vi "FF+FB control (Rev.2).vi"() -> ()   [LabVIEW 2010]
uses:
  <vilib>/DAQmx/read.llb/DAQmx Read (Analog 1D DBL NChan 1Samp).vi
  <vilib>/DAQmx/write.llb/DAQmx Write (Analog DBL 1Chan 1Samp).vi
  <vilib>/DAQmx/create/channels.llb/DAQmx Create Channel (AI-Voltage-Basic).vi
  <vilib>/DAQmx/configure/timing.llb/DAQmx Timing (Sample Clock).vi
  <vilib>/DAQmx/create/channels.llb/DAQmx Create Channel (AO-Voltage-Basic).vi
  <vilib>/daqmx/miscellaneous.llb/DAQmx Fill In Error Info.vi
panel:
  in  "ch2-1估測DC時間(秒)":dbl=1.0
  in  "ch2-2 估測DC時間(秒)":dbl=0.75
  in  "ch2 Kii 增益":dbl=-60000.0
  in  "ch2 Kp 增益":dbl
  out "overload":bool
  in  "ch1 Kp 增益":dbl=-250.0
  in  "ch2 Ki 增益":dbl=-83.5
  in  "ch1 Ki 增益":dbl=-10000.0
  in  "ch1-2估測DC時間(秒)":dbl=1.0
  in  "ch2-3估測DC時間(秒)":dbl=0.5
  in  "Controller on":bool
  out "error out":errorcluster
  out "延遲百分比(%)  需小於0.5%":dbl=0.3028175195295191
  out "理想迴圈時間(ms)":dbl=0.14285714285714288
  out "迴圈平均運行時間(ms)":dbl=0.14328973931361363
  in  "output channels 1":tag="PXI-6733/ao0"
  in  "stop":bool
  in  "ch1-1估測DC時間(秒)":dbl=2.0
  in  "每通道取樣頻率(Hz)":dbl=7000.0 format="%0.2f"
  in  "input channels 2":tag="PXI-6229/ai1"
  in  "input channels 1":tag="PXI-6229/ai0"
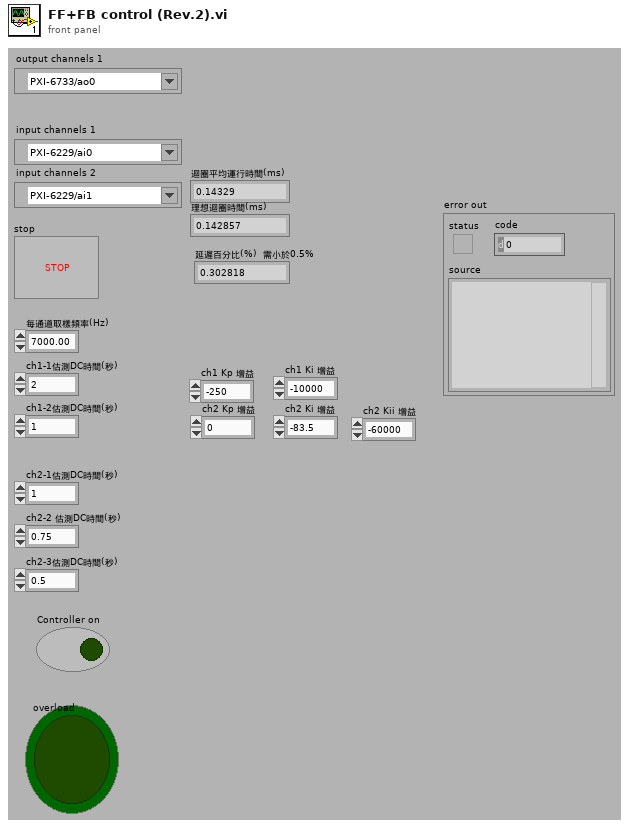
[diagram p1: front panel]
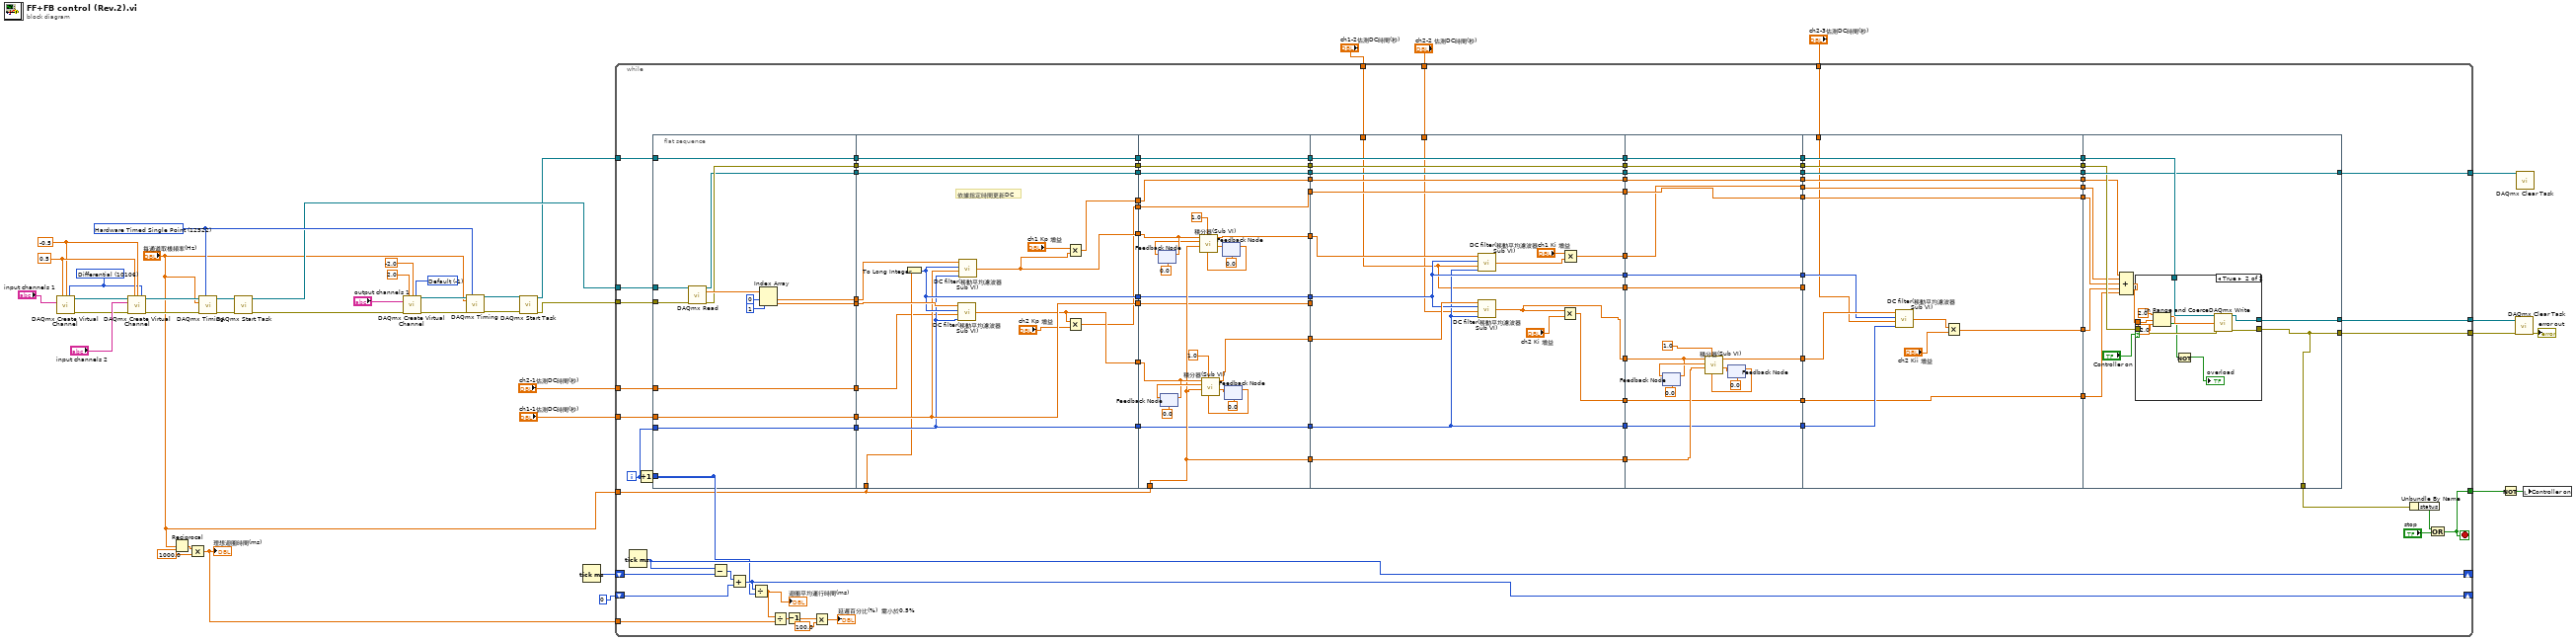
[diagram p0: block diagram]
diagram:
  w28 = -1 items=["Default"=-1, "RSE"=10083, "Differential"=10106, "Pseudodifferential"=12529] ("output terminal configuration")
  w25 = 12522 items=["Finite Samples"=10178, "Continuous Samples"=10123, "Hardware Timed Single Point"=12522] ("sample mode")
  w36 = 10106 items=["default"=-1, "RSE"=10083, "NRSE"=10078, "Differential"=10106, "Pseudodifferential"=12529] ("input terminal configuration")
  w37 = -0.5 ("minimum value")
  w38 = 0.5 ("maximum value")
  n1 = call-poly <vilib>:"DAQmx Create Virtual Channel.vi"("maximum value"=w38, "minimum value"=w37, "input terminal configuration"=w36, "physical channels"="input channels 1") -> ("task out"=w41:refnum<k21>, "error out"=w33:errorcluster)  [unwired: 10 in]
  n2 = call-poly <vilib>:"DAQmx Create Virtual Channel.vi"("task in"=w41, "maximum value"=w38, "minimum value"=w37, "input terminal configuration"=w36, "physical channels"="input channels 2", "error in"=w33) -> ("task out"=w35:refnum<k21>, "error out"=w32:errorcluster)  [unwired: 8 in]
  n3 = Reciprocal(x="每通道取樣頻率(Hz)") -> (1/x=w16:dbl)
  n4 = Multiply(x=w16, y=1000.0) -> (x*y=w14:dbl)
  "理想迴圈時間(ms)" <- w14
  n5 = call-poly <vilib>:"DAQmx Timing.vi"("task/channels in"=w35, "sample mode"=w25, "rate"="每通道取樣頻率(Hz)", "error in"=w32) -> ("task out"=w34:refnum<k21>, "error out"=w31:errorcluster)  [unwired: 10 in]
  n6 = call <vilib>:"DAQmx Start Task.vi"("task/channels in"=w34, "error in"=w31) -> ("task out"=w21:refnum<k21>, "error out"=w22:errorcluster)  [unwired: 12 in]
  n7 = call-poly <vilib>:"DAQmx Create Virtual Channel.vi"("maximum value"=2.0, "minimum value"=-2.0 ("maximum value"), "output terminal configuration"=w28, "physical channels"="output channels 1", "error in"=w22) -> ("task out"=w27:refnum<k21>, "error out"=w26:errorcluster)  [unwired: 9 in]
  n8 = call-poly <vilib>:"DAQmx Timing.vi"("task/channels in"=w27, "sample mode"=w25, "rate"="每通道取樣頻率(Hz)", "error in"=w26) -> ("task out"=w24:refnum<k21>, "error out"=w23:errorcluster)  [unwired: 10 in]
  n9 = call <vilib>:"DAQmx Start Task.vi"("task/channels in"=w24, "error in"=w23) -> ("task out"=w12:refnum<k21>, "error out"=w20:errorcluster)  [unwired: 12 in]
  n10 = Tick Count (ms)() -> (millisecond timer value=w18:u32)
  n11 = while {
    tunnel: w21 -> [w130]
    tunnel: w20 -> [w129]
    shift-right: [w125] -> _
    shift-left: w18 -> [w126]
    shift-right: [w122] -> _
    shift-left: 0 ("index") -> [w123]
    tunnel: w14 -> [w119]
    tunnel: "每通道取樣頻率(Hz)" -> [w69]
    tunnel: w12 -> [w106]
    tunnel: [w99] -> w9
    tunnel: [w67] -> w8
    tunnel: [w86] -> w7
    tunnel: "ch1-1估測DC時間(秒)" -> [w85]
    tunnel: [w68] -> w5
    tunnel: "ch1-2估測DC時間(秒)" -> [w46]
    tunnel: "ch2-3估測DC時間(秒)" -> [w45]
    tunnel: "ch2-2 估測DC時間(秒)" -> [w44]
    tunnel: "ch2-1估測DC時間(秒)" -> [w43]
    i -> [w83]
    stop <- w68 stop-if-true
    n12 = Tick Count (ms)() -> (millisecond timer value=w125:u32)
    n13 = Increment(x=w83) -> (x+1=w121:i32)
    n14 = flat-sequence {
      tunnel: w130 -> [w143]
      tunnel: w129 -> [w142]
      tunnel: [w138] -> w128
      tunnel: [w137] -> w127
      tunnel: w121 -> [_]
      tunnel: w106 -> [w136]
      tunnel: [w136] -> w100
      tunnel: [w135] -> w98
      tunnel: [w134] -> w92
      tunnel: w85 -> [w133]
      tunnel: [w133] -> w84
      tunnel: w83 -> [w132]
      tunnel: [w132] -> w82
      tunnel: w43 -> [w131]
      tunnel: [w131] -> w42
      tunnel: w128 -> [w156]
      tunnel: w127 -> [w155]
      tunnel: [w146] -> w114
      tunnel: [w149] -> w113
      tunnel: [w159] -> w101
      tunnel: w100 -> [w159]
      tunnel: w98 -> [w158]
      tunnel: [w158] -> w97
      tunnel: w92 -> [w157]
      tunnel: [w157] -> w87
      tunnel: w84 -> [w153]
      tunnel: w82 -> [w152]
      tunnel: [w154] -> w80
      tunnel: [w153] -> w79
      tunnel: [w152] -> w76
      tunnel: w69 -> [w151]
      tunnel: [w148] -> w59
      tunnel: [w145] -> w54
      tunnel: w42 -> [w144]
      tunnel: w114 -> [w173]
      tunnel: w113 -> [w184]
      tunnel: w69 -> [w170]
      tunnel: [w172] -> w112
      tunnel: [w171] -> w111
      tunnel: [w170] -> w108
      tunnel: [w169] -> w102
      tunnel: w101 -> [w169]
      tunnel: w97 -> [w168]
      tunnel: [w168] -> w95
      tunnel: [w167] -> w88
      tunnel: w87 -> [w167]
      tunnel: [w166] -> w81
      tunnel: w80 -> [w166]
      tunnel: w79 -> [w165]
      tunnel: [w165] -> w78
      tunnel: [w164] -> w77
      tunnel: w76 -> [w164]
      tunnel: w59 -> [w161]
      tunnel: [w161] -> w55
      tunnel: w54 -> [w160]
      tunnel: [w160] -> w53
      tunnel: w112 -> [w198]
      tunnel: w111 -> [w197]
      tunnel: [w190] -> w110
      tunnel: [w202] -> w109
      tunnel: w108 -> [w202]
      tunnel: [w201] -> w103
      tunnel: w102 -> [w201]
      tunnel: [w200] -> w96
      tunnel: w95 -> [w200]
      tunnel: [w199] -> w89
      tunnel: w88 -> [w199]
      tunnel: w81 -> [w196]
      tunnel: w78 -> [_]
      tunnel: w77 -> [w195]
      tunnel: [w196] -> w74
      tunnel: [w186] -> w72
      tunnel: [w195] -> w70
      tunnel: [w192] -> w56
      tunnel: w55 -> [w192]
      tunnel: w53 -> [w191]
      tunnel: [w191] -> w50
      tunnel: [w189] -> w48
      tunnel: [w188] -> w47
      tunnel: w46 -> [w186]
      tunnel: w44 -> [w185]
      tunnel: w110 -> [w207]
      tunnel: w109 -> [w216]
      tunnel: [w215] -> w107
      tunnel: [w214] -> w104
      tunnel: w103 -> [w214]
      tunnel: w96 -> [w213]
      tunnel: [w213] -> w93
      tunnel: [w212] -> w90
      tunnel: w89 -> [w212]
      tunnel: [w211] -> w75
      tunnel: w74 -> [w211]
      tunnel: [w210] -> w73
      tunnel: w72 -> [w210]
      tunnel: [w209] -> w71
      tunnel: w70 -> [w209]
      tunnel: [w203] -> w63
      tunnel: [w204] -> w60
      tunnel: [w206] -> w57
      tunnel: w56 -> [w206]
      tunnel: [w205] -> w51
      tunnel: w50 -> [w205]
      tunnel: w48 -> [w204]
      tunnel: w47 -> [w203]
      tunnel: w107 -> [w232]
      tunnel: [w235] -> w105
      tunnel: w104 -> [w235]
      tunnel: [w234] -> w94
      tunnel: w93 -> [w234]
      tunnel: [w233] -> w91
      tunnel: w90 -> [w233]
      tunnel: w75 -> [w231]
      tunnel: w73 -> [_]
      tunnel: w71 -> [w230]
      tunnel: w63 -> [w229]
      tunnel: [w229] -> w62
      tunnel: [w228] -> w61
      tunnel: w60 -> [w228]
      tunnel: [w227] -> w58
      tunnel: w57 -> [w227]
      tunnel: [w226] -> w52
      tunnel: w51 -> [w226]
      tunnel: [w223] -> w49
      tunnel: w45 -> [w222]
      tunnel: w105 -> [w247]
      tunnel: [w246] -> w99
      tunnel: w94 -> [w243]
      tunnel: [w242] -> w67
      tunnel: [w245] -> w86
      tunnel: w91 -> [w245]
      tunnel: [w242] -> w66
      tunnel: w62 -> [w239]
      tunnel: w61 -> [w236]
      tunnel: w58 -> [w240]
      tunnel: w52 -> [w238]
      tunnel: w49 -> [w237]
      frame #0 {
        n15 = call-poly <vilib>:"DAQmx Read.vi"("task/channels in"=w143, "error in"=w142) -> ("task out"=w134:refnum<k21>, "data"=w139:dbl[], "error out"=w135:errorcluster)  [unwired: 11 in]
        n16 = Index Array(array=w139, index #1=0 ("index"), index #2=1 ("index")) -> (element #1=w138:dbl, element #2=w137:dbl)
      }
      frame #1 {
        # "依據指定時間更新DC"
        n17 = To Long Integer(number=w151) -> (32bit integer=w154:i32)
        n18 = call "DC filter(移動平均濾波器 Sub VI).vi"("當前迴圈計數(i)"=w152, "平均時間"=w144, "取樣頻率(Hz)"=w154, "input signal"=w155) -> ("DC filter output"=w146:dbl)
        n19 = call "DC filter(移動平均濾波器 Sub VI).vi"("當前迴圈計數(i)"=w152, "平均時間"=w153, "取樣頻率(Hz)"=w154, "input signal"=w156) -> ("DC filter output"=w149:dbl)
        n20 = Multiply(x="ch1 Kp 增益", y=w149) -> (x*y=w148:dbl)
        n21 = Multiply(x=w146, y="ch2 Kp 增益") -> (x*y=w145:dbl)
      }
      frame #2 {
        n22 = feedback #1(0.0) -> (w183:dbl)
        n23 = feedback-in #1(w184) -> ()
        n24 = feedback #2(0.0) -> (w174:dbl)
        n25 = feedback-in #2(w173) -> ()
        n26 = feedback #3(0.0 ("輸出累加ERR回朔")) -> (w181:dbl)
        n27 = call "積分器(Sub VI).vi"("輸入累加ERR回朔"=w181, "I增益"=1.0, "samples (Hz)"=w170, "前一個ERR"=w183, "當下ERR"=w184) -> ("輸出累加ERR回朔"=w182:dbl, "積分修正量"=w172:dbl)  [unwired: 5 in]
        n28 = feedback-in #3(w182) -> ()
        n29 = feedback #4(0.0 ("輸出累加ERR回朔")) -> (w176:dbl)
        n30 = call "積分器(Sub VI).vi"("輸入累加ERR回朔"=w176, "I增益"=1.0, "samples (Hz)"=w170, "前一個ERR"=w174, "當下ERR"=w173) -> ("輸出累加ERR回朔"=w175:dbl, "積分修正量"=w171:dbl)  [unwired: 5 in]
        n31 = feedback-in #4(w175) -> ()
      }
      frame #3 {
        n32 = call "DC filter(移動平均濾波器 Sub VI).vi"("當前迴圈計數(i)"=w195, "平均時間"=w186, "取樣頻率(Hz)"=w196, "input signal"=w198) -> ("DC filter output"=w187:dbl)
        n33 = call "DC filter(移動平均濾波器 Sub VI).vi"("當前迴圈計數(i)"=w195, "平均時間"=w185, "取樣頻率(Hz)"=w196, "input signal"=w197) -> ("DC filter output"=w190:dbl)
        n34 = Multiply(x=w190, y="ch2 Ki 增益") -> (x*y=w189:dbl)
        n35 = Multiply(x="ch1 Ki 增益", y=w187) -> (x*y=w188:dbl)
      }
      frame #4 {
        n36 = feedback #5(0.0) -> (w217:dbl)
        n37 = feedback-in #5(w207) -> ()
        n38 = feedback #6(0.0 ("輸出累加ERR回朔")) -> (w219:dbl)
        n39 = call "積分器(Sub VI).vi"("輸入累加ERR回朔"=w219, "I增益"=1.0, "samples (Hz)"=w216, "前一個ERR"=w217, "當下ERR"=w207) -> ("輸出累加ERR回朔"=w218:dbl, "積分修正量"=w215:dbl)  [unwired: 5 in]
        n40 = feedback-in #6(w218) -> ()
      }
      frame #5 {
        n41 = call "DC filter(移動平均濾波器 Sub VI).vi"("當前迴圈計數(i)"=w230, "平均時間"=w222, "取樣頻率(Hz)"=w231, "input signal"=w232) -> ("DC filter output"=w225:dbl)
        n42 = Multiply(x=w225, y="ch2 Kii 增益") -> (x*y=w223:dbl)
      }
      frame #6 {
        n43 = Compound Arithmetic op=ADD(w240, w239, w238, w237, w236) -> (w241:dbl)
        n44 = case shown="True" "Controller on" {
          tunnel: w247 -> [_ w257]
          tunnel: [_ w256] -> w246
          tunnel: w243 -> [_ w255]
          tunnel: [_ w254] -> w242
          tunnel: w241 -> [_ w253]
          frame False {
          }
          frame True {
            n45 = In Range and Coerce(upper limit=2.0, x=w253, lower limit=-2.0) -> (coerced(x)=w252:dbl, In Range?=w249:bool)
            n46 = Not(x=w249) -> (.not. x?=→"overload":bool)
            n47 = call-poly <vilib>:"DAQmx Write.vi"("task/channels in"=w257, "data"=w252, "error in"=w255) -> ("task out"=w256:refnum<k21>, "error out"=w254:errorcluster)  [unwired: 10 in, 1 out]
          }
        }
      }
    }
    n48 = Subtract(x=w125, y=w126) -> (x-y=w124:u32)
    n49 = Add(x=w124, y=w123) -> (x+y=w122:u32)
    n50 = Divide(x=w122, y=w121) -> (x/y=w120:dbl)
    "迴圈平均運行時間(ms)" <- w120
    n51 = Divide(x=w120, y=w119) -> (x/y=w118:dbl)
    n52 = Decrement(x=w118) -> (x-1=w117:dbl)
    n53 = Multiply(x=w117, y=100.0) -> (x*y=→"延遲百分比(%)  需小於0.5%":dbl)
    n54 = Unbundle By Name(w66) -> ("status"=w65:bool)
    n55 = Or(x=w65, y="stop") -> (x .or. y?=w68:bool)
  }
  n56 = Not(x=w5) -> (.not. x?=w6:bool)
  n57 = call <vilib>:"DAQmx Clear Task.vi"("task in"=w9, "error in"=w8) -> ("error out"=→"error out":errorcluster)  [unwired: 13 in]
  n58 = call <vilib>:"DAQmx Clear Task.vi"("task in"=w7) -> ()  [unwired: 14 in, 1 out]
  n59 = local write "Controller on"(w6) -> ()
